vi "ma_SML ND Zoom FFT.vi"   [LabVIEW 2020, in "NI_MAPro.lvlib"]
uses:
  NI_MAPro.lvlib
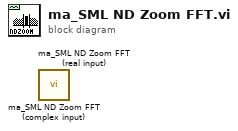
[diagram p0: block diagram]
diagram:
  n1 = call "ma_SML ND Zoom FFT (complex input).vi"() -> ()  [unwired: 5 in, 3 out]
  n2 = call "ma_SML ND Zoom FFT (real input).vi"() -> ()  [unwired: 5 in, 3 out]
